vi "Get System Events.vi"(8 "error in (no error)":errorcluster) -> (0 "error out":errorcluster, 3 "system events":cluster{"timestamp":string, "message":string}[](array[cluster]))   [LabVIEW 2023]
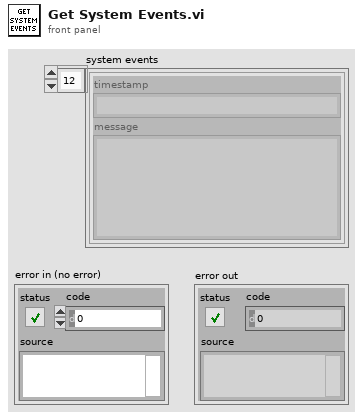
[diagram p1: front panel]
types:
  T1 = enum16{"open", "replace", "create", "open or create", "replace or create", "replace or create with confirmation"}
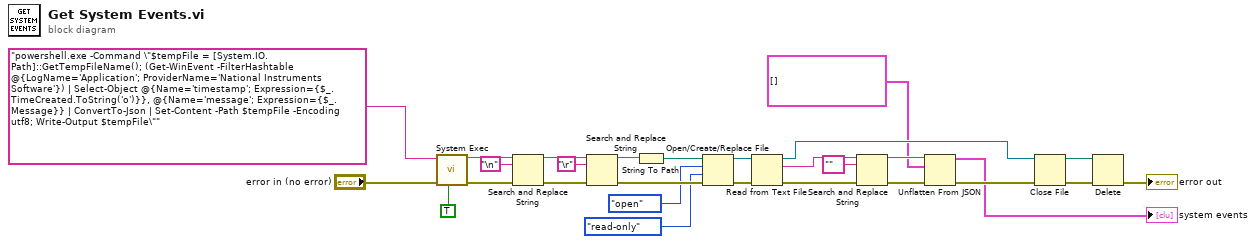
[diagram p0: block diagram]
diagram:
  n1 = call <vilib>:"System Exec.vi"("run minimized? (F)"=TRUE, "error in (no error)"="error in (no error)", "command line"="powershell.exe -Command \"$tempFile = [System.IO.Path]::GetTempFileName(); (Get-WinEvent -FilterHashtable @{LogName='Application'; ProviderName='National Instruments Software'}) | Select-Object @{Name='timestamp'; Expression={$_.TimeCreated.ToString('o')}}, @{Name='message'; Expression={$_.Message}} | ConvertTo-Json | Set-Content -Path $tempFile -Encoding utf8; Write-Output $tempFile\"" ("format string")) -> ("error out"=w20:errorcluster, "standard output"=w15:string)  [unwired: 5 in, 2 out]
  n2 = Search and Replace String(input string=w15, search string="\n", error in=w20) -> (result string=w16:string, error out=w19:errorcluster)  [unwired: 5 in, 2 out]
  n3 = Search and Replace String(input string=w16, search string="\r", error in=w19) -> (result string=w17:string, error out=w18:errorcluster)  [unwired: 5 in, 2 out]
  n4 = String To Path(string=w17) -> (path=w22:path)
  n5 = Open/Create/Replace File(file path (use dialog)=w22, error in=w18, operation (0:open)=T1."open", access (0:read/write)=enum16{"read/write", "read-only", "write-only"}."read-only") -> (refnum out=w25:refnum<file>, error out=w26:errorcluster)  [unwired: 2 in, 1 out]
  n6 = Read from Text File(file (use dialog)=w25, error in=w26) -> (refnum out=w4:refnum<file>, text=w9:string, error out=w10:errorcluster)  [unwired: 2 in, 1 out]
  n7 = Search and Replace String(input string=w9, search string="﻿", error in=w10) -> (result string=w7:string, error out=w6:errorcluster)  [unwired: 5 in, 2 out]
  n8 = Unflatten From JSON(JSON string=w7, type and defaults=cluster{"timestamp":string, "message":string}[] [], error in (no error)=w6) -> (value=→"system events":cluster{"timestamp":string, "message":string}[], error out=w5:errorcluster)  [unwired: 4 in]
  n9 = Close File(refnum=w4, error in=w5) -> (path=w23:path, error out=w24:errorcluster)
  n10 = Delete(path (use dialog)=w23, error in=w24) -> (error out=→"error out":errorcluster)  [unwired: 3 in, 2 out]
